vi "NI6008 Enout Trigger.vi"(8 "error in (no error)":errorcluster, 11 "Actor_NI6008 in":refnum<class "Actor_NI6008.lvclass">) -> (0 "error out":errorcluster, 3 "Actor_NI6008 out":refnum<class "Actor_NI6008.lvclass">)   [LabVIEW 2020, in "Actor_NI6008.lvlib" / "Actor_NI6008.lvclass"]
uses:
  Actor_NI6008.lvclass
  C:/Program Files/National Instruments/LabVIEW 2020/vi.lib/ActorFramework/Actor/Actor.lvclass
  <vilib>/ActorFramework/Actor/Actor.lvclass/Actor.ctl
  Actor_NI6008.lvclass/Actor_NI6008.ctl
  I_NI6008 Messages/NI6008 Status Report Msg/NI6008 Status Report Msg.lvclass/NI6008 Status Report Msg.ctl
  <vilib>/ActorFramework/Message Enqueuer/Message Enqueuer.lvclass/Message Enqueuer.ctl
  <vilib>/DAQmx/write.llb/DAQmx Write (Digital Bool 1Line 1Point).vi
  <vilib>/ActorFramework/Message Enqueuer/Enqueue.vi
  I_NI6008 Messages/NI6008 Status Report Msg/NI6008 Status Report Msg.lvclass
  C:/Program Files/National Instruments/LabVIEW 2020/vi.lib/ActorFramework/Message/Message.lvclass
  <vilib>/DAQmx/miscellaneous.llb/DAQmx Fill In Error Info.vi
  <vilib>/ActorFramework/Message Priority Queue/Priority Enqueue.vi
  <vilib>/ActorFramework/Actor/Actor.lvclass
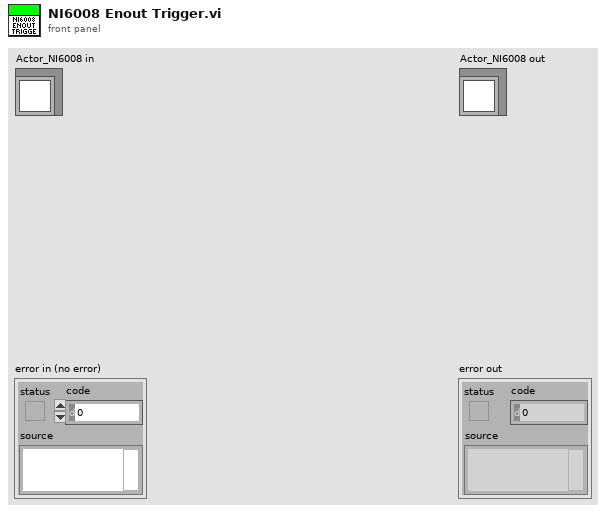
[diagram p1: front panel]
types:
  T1 = cluster{"Msg":string, "DO":bool[], "AI":dbl, "NI6008 Error":errorcluster}
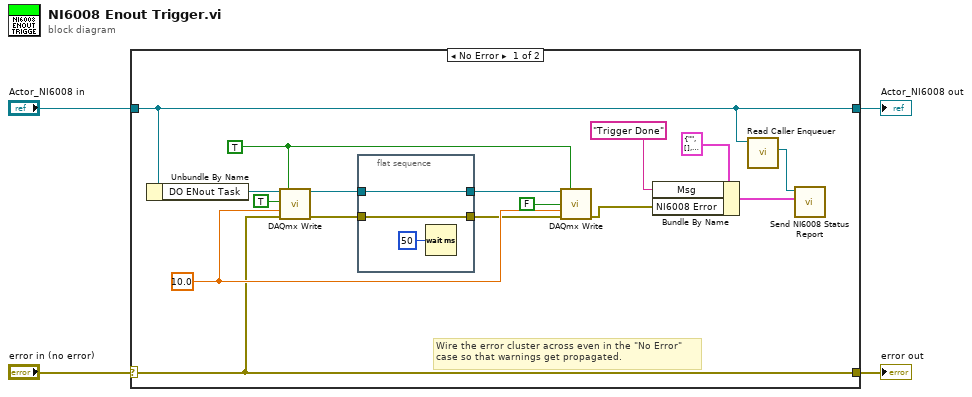
[diagram p0: block diagram]
diagram:
  n1 = case shown="No Error" "error in (no error)" {
    selector: "error in (no error)" -> [w11 w25]
    tunnel: [w11 w25] -> w3
    tunnel: [w16 w24] -> w1
    tunnel: "Actor_NI6008 in" -> [w16 w24]
    frame No Error {
      w12 = TRUE ("auto start")
      w13 = 10.0 ("timeout")
      # "Wire the error cluster across even in the \"No Error\"\ncase so that warnings get propagated."
      n2 = Unbundle By Name(w16) -> ("DO ENout Task"=w15:refnum<k21>)
      n3 = call-poly <vilib>:"DAQmx Write.vi"("task/channels in"=w15, "auto start"=w12, "data"=TRUE, "timeout"=w13, "error in"=w11) -> ("task out"=w8:refnum<k21>, "error out"=w6:errorcluster)  [unwired: 8 in, 1 out]
      n4 = flat-sequence {
        tunnel: w8 -> [w23]
        tunnel: [w23] -> w7
        tunnel: w6 -> [w22]
        tunnel: [w22] -> w5
        frame #0 {
          n5 = Wait (ms)(milliseconds to wait=u32 50) -> ()  [unwired: 1 out]
        }
      }
      n6 = call-poly <vilib>:"DAQmx Write.vi"("task/channels in"=w7, "auto start"=w12, "data"=FALSE, "timeout"=w13, "error in"=w5) -> ("error out"=w14:errorcluster)  [unwired: 8 in, 2 out]
      n7 = Bundle By Name(cluster=T1 {"Msg"="", "DO"=[], "AI"=0.0, "NI6008 Error"={"status"=FALSE, "code"=0, "source"=""}} ("Data"), "Msg"="Trigger Done", "NI6008 Error"=w14) -> (w18:T1)
      n8 = call <vilib>:"Read Caller Enqueuer.vi"("Actor"=w16) -> ("Caller Enqueuer"=w17:refnum<class "Message Enqueuer.lvclass">)  [unwired: 10 in]
      n9 = call "Send NI6008 Status Report.vi"("Data"=w18, "Message Enqueuer"=w17) -> ()  [unwired: 8 in, 2 out]
    }
    frame Error {
    }
  }
  "error out" <- w3
  "Actor_NI6008 out" <- w1
